vi "get duplicate file in specific folders.vi"(11 "All Folders":path[](array[path])) -> (3 "Array":path[](array[path]))   [LabVIEW 2023]
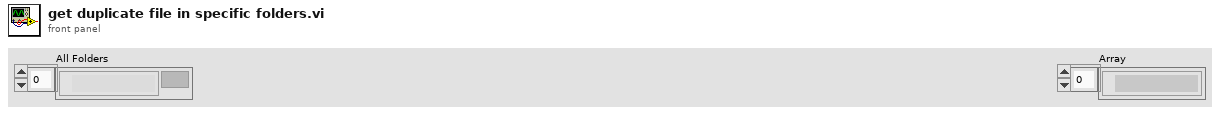
[diagram p1: front panel]
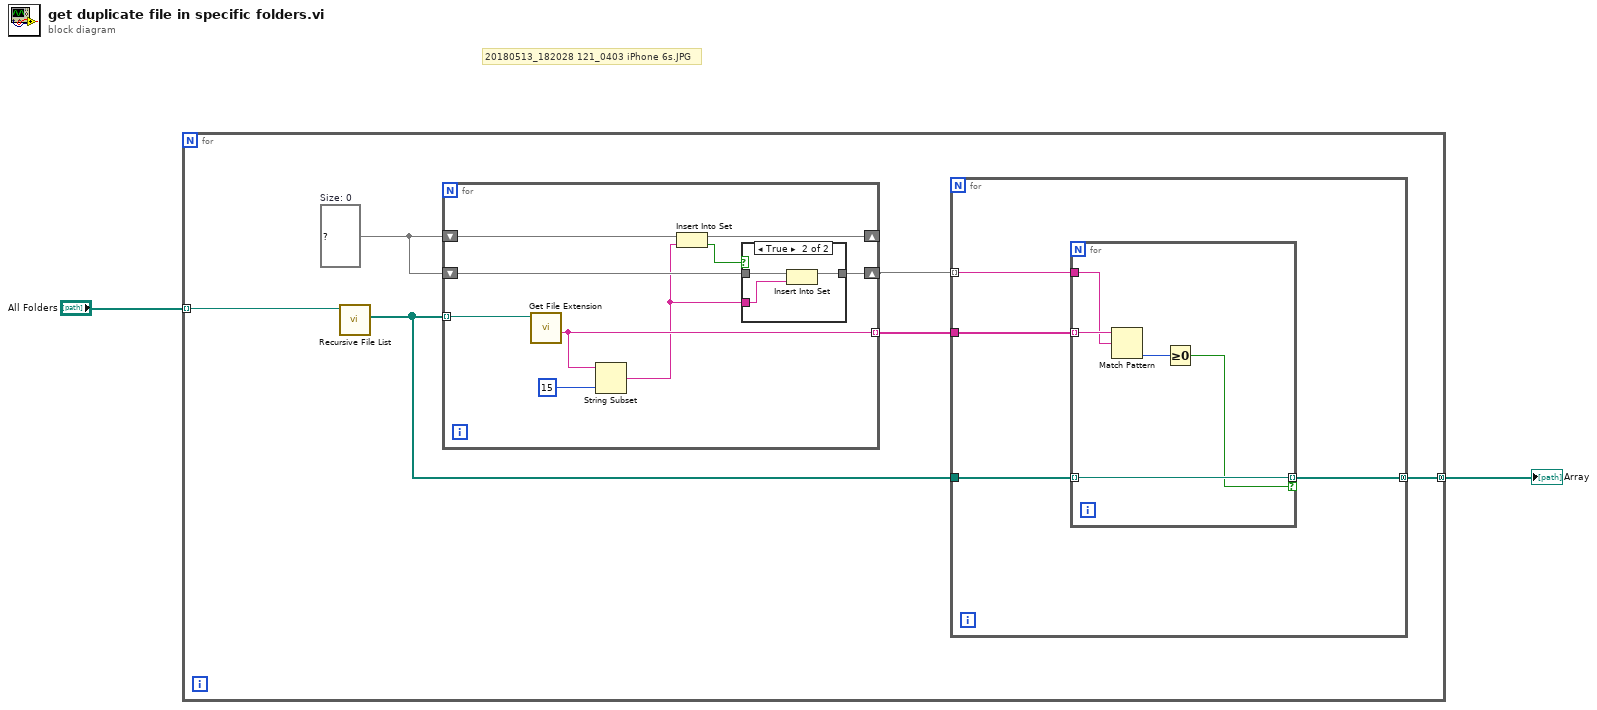
[diagram p0: block diagram]
diagram:
  # "20180513_182028 121_0403 iPhone 6s.JPG"
  n1 = for {
    tunnel: "All Folders" -> [w8] mode=indexing
    tunnel: [w5] -> w1 mode=concatenating
    w4 = set{string} {}  # Size: 0
    n2 = call <vilib>:"Recursive File List.vi"("Folder Path"=w8) -> ("All Files in Dir"=w6:path[])  [unwired: 6 in, 4 out]
    n3 = for {
      tunnel: w6 -> [w26] mode=indexing
      shift-right: [w23] -> _
      shift-left: w4 -> [w24]
      tunnel: [w22] -> w7 mode=indexing
      shift-right: [w21] -> w3
      shift-left: w4 -> [w19]
      n4 = call <vilib>:"Get File Extension.vi"("file"=w26) -> ("filename without extension"=w22:string)  [unwired: 6 in, 4 out]
      n5 = String Subset(string=w22, length (rest)=15 ("length (rest)")) -> (substring=w18:string)  [unwired: 1 in]
      n6 = Insert Into Set(10:w18, 11:w24) -> (2:w20:bool, 3:w23:set{string})
      n7 = case shown="True" w20 {
        tunnel: [w27 w30] -> w21
        tunnel: w19 -> [w27 w29]
        tunnel: w18 -> [_ w28]
        frame False {
        }
        frame True {
          n8 = Insert Into Set(10:w28, 11:w29) -> (3:w30:set{string})  [unwired: 1 out]
        }
      }
    }
    n9 = for {
      tunnel: w7 -> [w12]
      tunnel: w6 -> [w10]
      tunnel: [w11] -> w5 mode=concatenating
      tunnel: w3 -> [w9] mode=indexing
      n10 = for {
        tunnel: w12 -> [w17] mode=indexing
        tunnel: w9 -> [w16]
        tunnel: [w14] -> w11 mode=indexing if=w13
        tunnel: w10 -> [w14] mode=indexing
        n11 = Match Pattern(string=w17, regular expression=w16) -> (offset past match=w15:i32)  [unwired: 1 in, 3 out]
        n12 = Greater Or Equal To 0?(x=w15) -> (x >= 0?=w13:bool)
      }
    }
  }
  "Array" <- w1
